vi "Tell Self Forward.vi"(7 "Actor in":refnum<class "Actor.lvclass">, 8 "Error in":errorcluster, 10 "Msg Attributes":refnum<data-value>) -> (0 "Error out":errorcluster, 5 "Actor out":refnum<class "Actor.lvclass">)   [LabVIEW 2020, in "_Template.lvlib" / "Templates.lvlib" / "TEMPLATE jettl Msg.lvlib" / "TEMPLATE.lvlib"]
uses:
  TEMPLATE.lvlib
  jettl/jettl/jettl.lvlib
  TEMPLATE jettl Msg.lvlib
  jettl/jettl/Actor/Actor.lvclass
  jettl/jettl/Relation.ctl
  jettl/jettl/Teller.ctl
  jettl/jettl/Msg Input/Msg Input.lvclass
  jettl/jettl/Msg Output/Msg Output.lvclass
  jettl/jettl/Msg/Msg.lvclass
  jettl/jettl/Msg Attributes.ctl
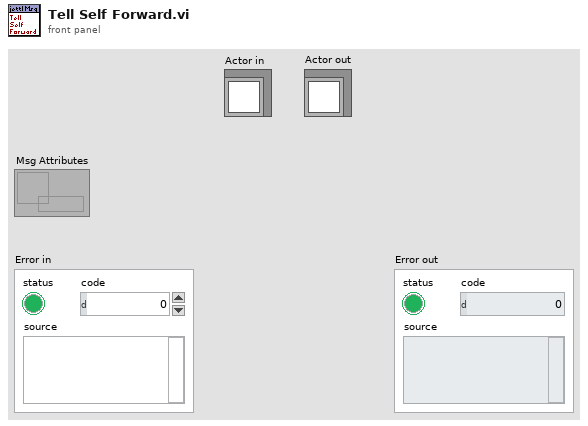
[diagram p1: front panel]
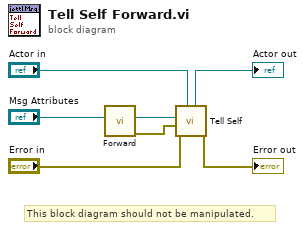
[diagram p0: block diagram]
diagram:
  # "This block diagram should not be manipulated."
  n1 = call "Forward.vi"("Msg Attributes in"="Msg Attributes") -> ("Error out"=w1:errorcluster, "Msg Attributes out"=w2:refnum<data-value>)  [unwired: 9 in]
  n2 = call "Tell Self.vi"("Actor in"="Actor in", "Error in"="Error in", "Error"=w1, "Msg Attributes"=w2) -> ("Error out"=→"Error out":errorcluster, "Actor out"=→"Actor out":refnum<class "Actor.lvclass">)  [unwired: 6 in]
